vi "Write Solution.vi"(8 "error in (no error)":errorcluster, 10 "Solution":T1[][](array[typedef]), 11 "Module Data in":refnum<class "Grassfire Algorithm.lvclass">) -> (0 "error out":errorcluster, 3 "Module Data out":refnum<class "Grassfire Algorithm.lvclass">)   [LabVIEW 2019, in "Grassfire Algorithm.lvclass"]
uses:
  Grassfire Algorithm.lvclass
  Solution Grid Cell--cluster.ctl
  Solution--picture ring.ctl
  Grassfire Algorithm.lvclass/Grassfire Algorithm.ctl
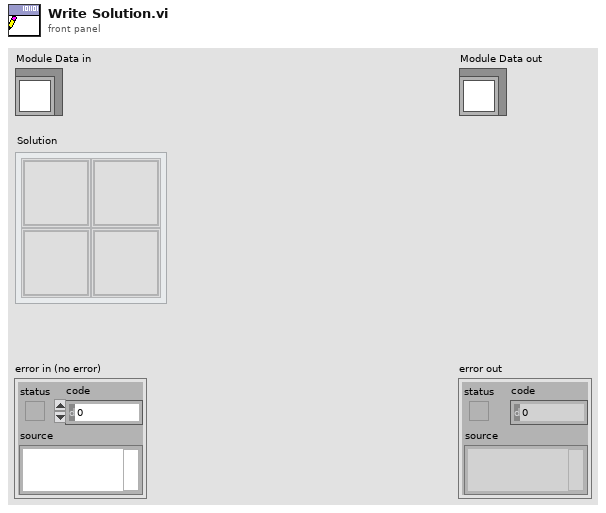
[diagram p1: front panel]
types:
  T1 = typedef "Grassfire Algorithm.lvclass/Solution Grid Cell--cluster.ctl" = cluster{"Picture":T2, "Value":string}
  T2 = typedef "Grassfire Algorithm.lvclass/Solution--picture ring.ctl" = i64
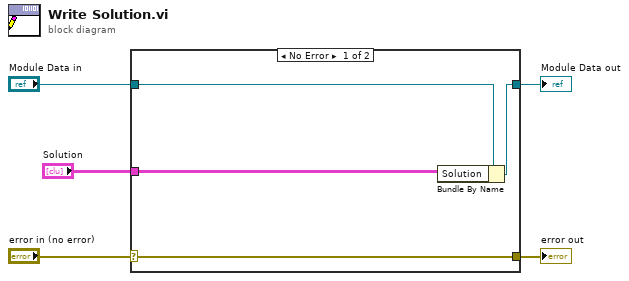
[diagram p0: block diagram]
diagram:
  n1 = case shown="No Error" "error in (no error)" {
    selector: "error in (no error)" -> [w9 w10]
    tunnel: [w9 w10] -> w4
    tunnel: [w7 w11] -> w2
    tunnel: "Module Data in" -> [w8 w11]
    tunnel: "Solution" -> [w6 _]
    frame No Error {
      n2 = Bundle By Name(cluster=w8, "Solution"=w6) -> (w7:refnum<class "Grassfire Algorithm.lvclass">)
    }
    frame Error {
    }
  }
  "error out" <- w4
  "Module Data out" <- w2
